vi "Configure Trigger Model Branch Counter Block.vi"(0 "VISA resource name":refnum<visa-resource-name>, 5 "Block Number (1)":i32=1 min=1 format="%#.6g", 7 "Branch Path (1)":i32=1 min=1 format="%#.6g", 9 "Target Count (1)":u32=1 min=1, 11 "error in (no error)":errorcluster) -> (4 "VISA resource name out":refnum<visa-resource-name>, 15 "error out":errorcluster)   [LabVIEW 2022 SP3, in "Keithley 2450.lvlib"]
doc: "This VI branches to a specified block a specified number of times."
uses:
  Keithley 2450.lvlib
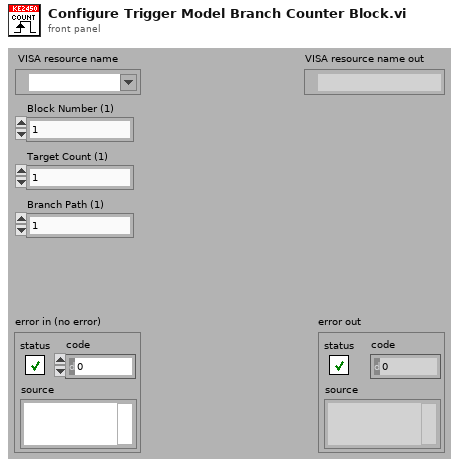
[diagram p1: front panel]
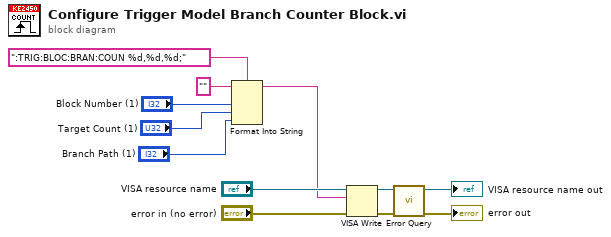
[diagram p0: block diagram]
diagram:
  n1 = Format Into String(format string=":TRIG:BLOC:BRAN:COUN %d,%d,%d;", initial string="", "Block Number (1)", "Target Count (1)", "Branch Path (1)") -> (resulting string=w3:string)  [unwired: 1 in, 1 out]
  n2 = VISA Write(VISA resource name="VISA resource name", write buffer=w3, error in (no error)="error in (no error)") -> (VISA resource name out=w8:refnum<visa-resource-name>, error out=w7:errorcluster)  [unwired: 1 out]
  n3 = call "Error Query.vi"("error in (no error)"=w7, "VISA resource name"=w8) -> ("error out"=→"error out":errorcluster, "VISA resource name out"=→"VISA resource name out":refnum<visa-resource-name>)  [unwired: 8 out]
